vi "Get Termination Status.vi"(8 "error in (no error)":errorcluster, 11 "Teststand in":refnum<class "Teststand.lvclass">) -> (0 "error out":errorcluster, 1 "Terminating or Aborting":bool, 3 "Teststand out":refnum<class "Teststand.lvclass">)   [LabVIEW 2023, in "HardwareAbstractionLayer_LVOOP.lvlib" / "Teststand.lvclass"]
uses:
  Teststand.lvclass
  Teststand.lvclass/Teststand.ctl
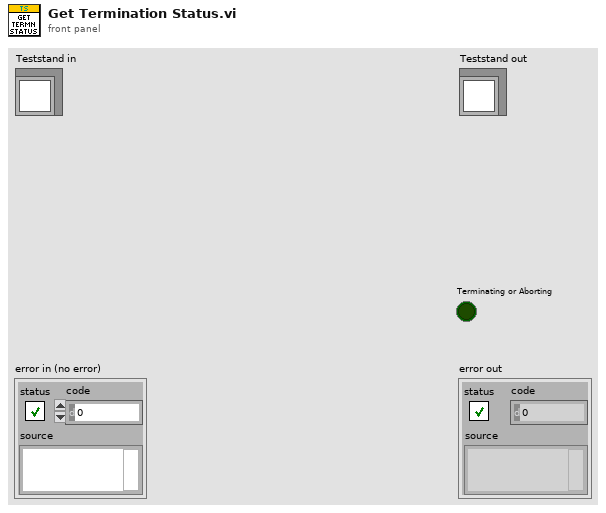
[diagram p1: front panel]
types:
  T1 = typedef "TestStand - Status Monitor.ctl" = cluster{"Sequence Context":refnum<k7>, "Execution":refnum<k7>, "Termination Monitor":refnum<k7>}
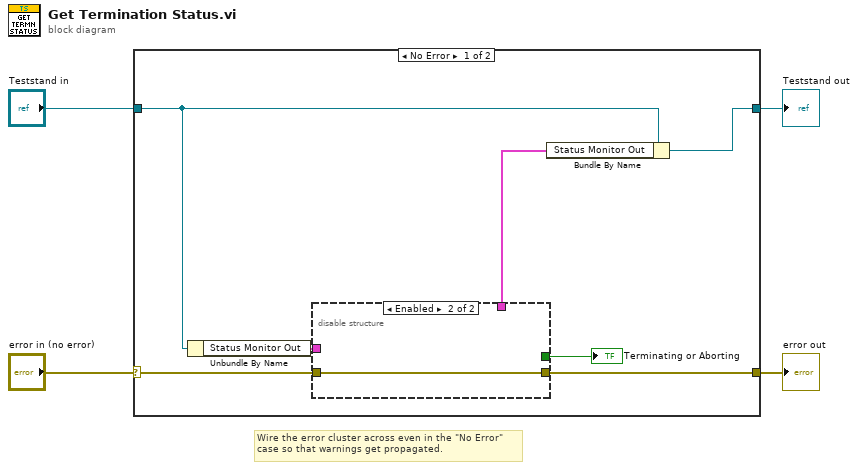
[diagram p0: block diagram]
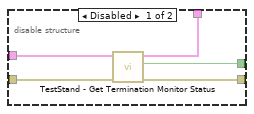
[diagram p2: hidden frame]
diagram:
  # "Wire the error cluster across even in the \"No Error\"\ncase so that warnings get propagated."
  n1 = case shown="No Error" "error in (no error)" {
    selector: "error in (no error)" -> [w11 w19]
    tunnel: [w10 w19] -> w3
    tunnel: [w5 w18] -> w1
    tunnel: "Teststand in" -> [w7 w18]
    frame No Error {
      n2 = Unbundle By Name(w7) -> ("Status Monitor Out"=w8:T1)
      n3 = disable-structure shown="Enabled" {
        disable-tunnel: w11 -> [w16 w17]
        disable-tunnel: [w15 w17] -> w10
        disable-tunnel: [w14 _] -> w9
        disable-tunnel: w8 -> [w13 _]
        disable-tunnel: [w12 _] -> w6
        frame Disabled {
          n4 = call <vilib>:"TestStand - Get Termination Monitor Status.vi"("error in (no error)"=w16, "Status Monitor In"=w13) -> ("error out"=w15:errorcluster, "Terminating or Aborting"=w14:bool, "Status Monitor Out"=w12:T1)  [unwired: 7 in]
        }
        frame Enabled {
        }
      }
      "Terminating or Aborting" <- w9
      n5 = Bundle By Name(cluster=w7, "Status Monitor Out"=w6) -> (w5:refnum<class "Teststand.lvclass">)
    }
    frame Error {
    }
  }
  "error out" <- w3
  "Teststand out" <- w1
